vi "IT7800 Driver Test.vi"() -> ()   [LabVIEW 2025]
uses:
  <vilib>/Platform/TimedLoop/XDataNode/timing_clust.ctl
  <vilib>/Platform/TimedLoop/XDataNode/nitl_modes.ctl
  <vilib>/Platform/TimedLoop/XDataNode/wakeup.ctl
  TypeDefs/CMD - Control.ctl
  <vilib>/Platform/TimedLoop/XDataNode/XDataNode.xnode
  <vilib>/Platform/TimedLoop/XDataNode/XDNodeRunTimeDep.lvlib
  <instrlib>/IT7800/IT7800.lvlib
panel:
  in  "CLR Error":bool
  out "Error":string
  in  "Tabs":enum32{"Testing", "Commands"}(tab)
  out "ValRead":bool
  in  "ReadInfo":bool
  in  "Command":T1(ring)
  in  "Write":bool
  in  "Parameter":dbl=50.0
  out "Output ON":bool
  out "Phase Config":string="-"
  in  "Read":bool=TRUE
  out "PSU Values":T2
  out "IT7800 Info":T3
  out "PSU Values 3PH":T4
  in  "String":string="FETC:VOLT?;\\s:FETC:FREQ?;\\s:FETC:CURR?;\\s:FETC:CURR:CFAC?;\\s:FETC:LTLV?\\sBA\n\nFETC:POW:REAL?;\\sPOW:APP?;\\s:FETC:POW:REAC?;\\sPOW:PFAC?\n\nFETC:WHO:ACT:POS?;\\s:FETC:WHO:ACT:NEG?"
  in  "SendCMD":bool
  out "Response":string
  in  "Request":string="FETC:VOLT?; :FETC:FREQ?"
  out "Open string":string
  in  "Exit":bool
  out "COM":bool
  in  "Close COM":bool
  in  "Open COM":bool
  in  "PSU Address":refnum<visa-resource-name>="192.168.0.252"
  # "Note: Change pase configuration only when output OFF"
  # "Note: In 3phase system PSU values are averages from 3Phases"
  # "Other examples used in software..."
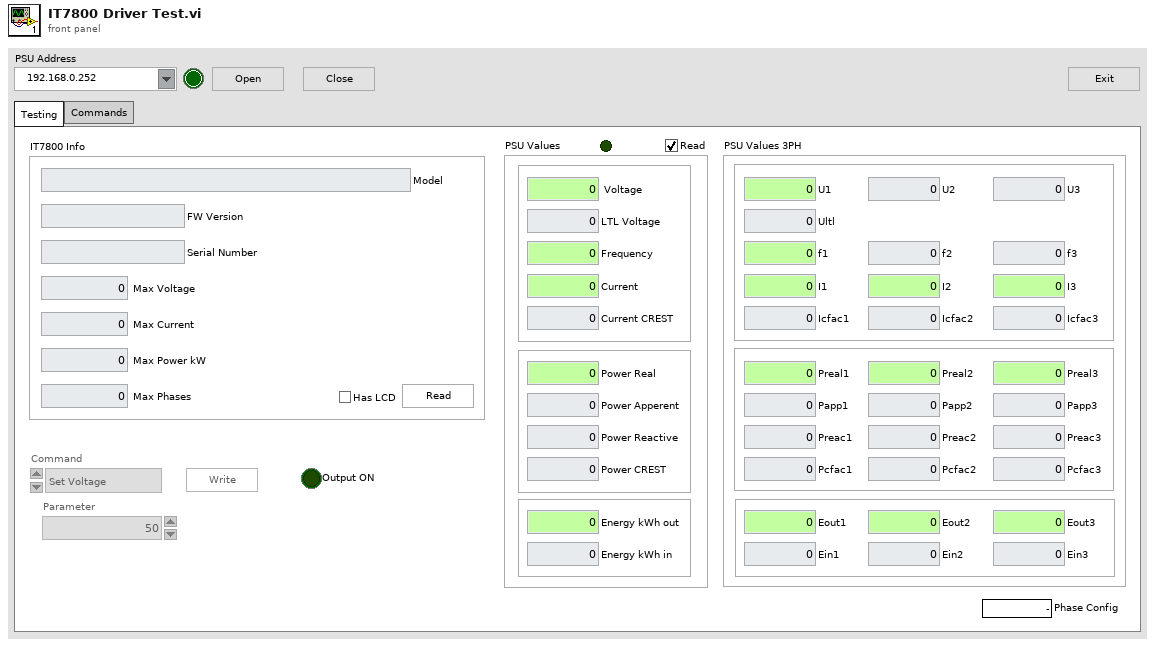
[diagram p1: front panel]
types:
  T1 = enum16{"Set Voltage", "Set Frequency", "Set to 1Phase", "Set to 3Phase", "Set to Split Phase", "Output ON", "Output OFF"}
  T2 = cluster{"Voltage":dbl, "LTL Voltage":dbl, "Current":dbl, "Current CREST":dbl, "Power Real":dbl, "Power Apperent":dbl, "Power Reactive":dbl, "Power CREST":dbl, "Energy kWh out":dbl, "Energy kWh in":dbl, "Frequency":dbl}
  T3 = cluster{"Model":string, "FW Version":string, "Serial Number":string, "Max Voltage":dbl, "Max Current":dbl, "Max Power kW":dbl, "Max Phases":u8, "Has LCD":bool}
  T4 = cluster{"U1":dbl, "U2":dbl, "U3":dbl, "Ultl":dbl, "f1":dbl, "f2":dbl, "f3":dbl, "I1":dbl, "I2":dbl, "I3":dbl, "Icfac1":dbl, "Icfac2":dbl, "Icfac3":dbl, "Preal1":dbl, "Preal2":dbl, "Preal3":dbl, "Papp1":dbl, "Papp2":dbl, "Papp3":dbl, "Preac1":dbl, "Preac2":dbl, "Preac3":dbl, "Pcfac1":dbl, "Pcfac2":dbl, "Pcfac3":dbl, "Eout1":dbl, "Eout2":dbl, "Eout3":dbl, "Ein1":dbl, "Ein2":dbl, "Ein3":dbl}
  T5 = enum32{"invalid app kind", "Development System", "Run Time System", "Student Edition", "Embedded LabVIEW", "Evaluation", "Custom"}
  T6 = enum8{"Enabled", "Disabled", "Disabled and Grayed Out"}
  T7 = typedef "XDNodeRunTimeDep.lvlib/timing_clust.ctl" = cluster{"Expected End [f-1]":u64, "Actual End [f-1]":u64, "Finished Late? [f-1]":bool, "Expected End [i-1]":u64, "Actual End [i-1]":u64, "Finished Late? [i-1]":bool, "Expected Start [i]":u64, "Actual Start [i]":u64, "Expected Start [f]":u64, "Actual Start [f]":u64, "Source Name":string, "Structure Name":string, "Period":i64, "Deadline":i64, "Offset":i64, "Start":i64, "Priority":i32, "Timeout":i32, "Mode":T8, "Wakeup Reason":T9, "Error":errorcluster, "Source Type":string, "Secondary Source Type":string, "Global End Time":u64, "Global Start Time":u64, "Frame Duration":u64, "Iteration Duration":u64, "Assigned CPU":i32, "I/O Scan Engine Mode":u32}
  T8 = typedef "XDNodeRunTimeDep.lvlib/nitl_modes.ctl" = enum32{"No Change", "Process missed periods, maintain original phase", "Discard missed periods, maintain original phase", "Process missed periods, ignore original phase", "Discard missed periods, ignore original phase"}
  T9 = typedef "XDNodeRunTimeDep.lvlib/wakeup.ctl" = enum32{"Normal", "Aborted", "Asynchronous wakeup", "Timing source error", "Timed loop error", "Timeout"}
  T10 = typedef "CMD - Control.ctl" = enum16{"Voltage", "Frquency", "Set Phases", "Output", "Measure Rate"}
  T11 = cluster{"Basic  quantities":bool, "Power":bool, "Energy":bool}
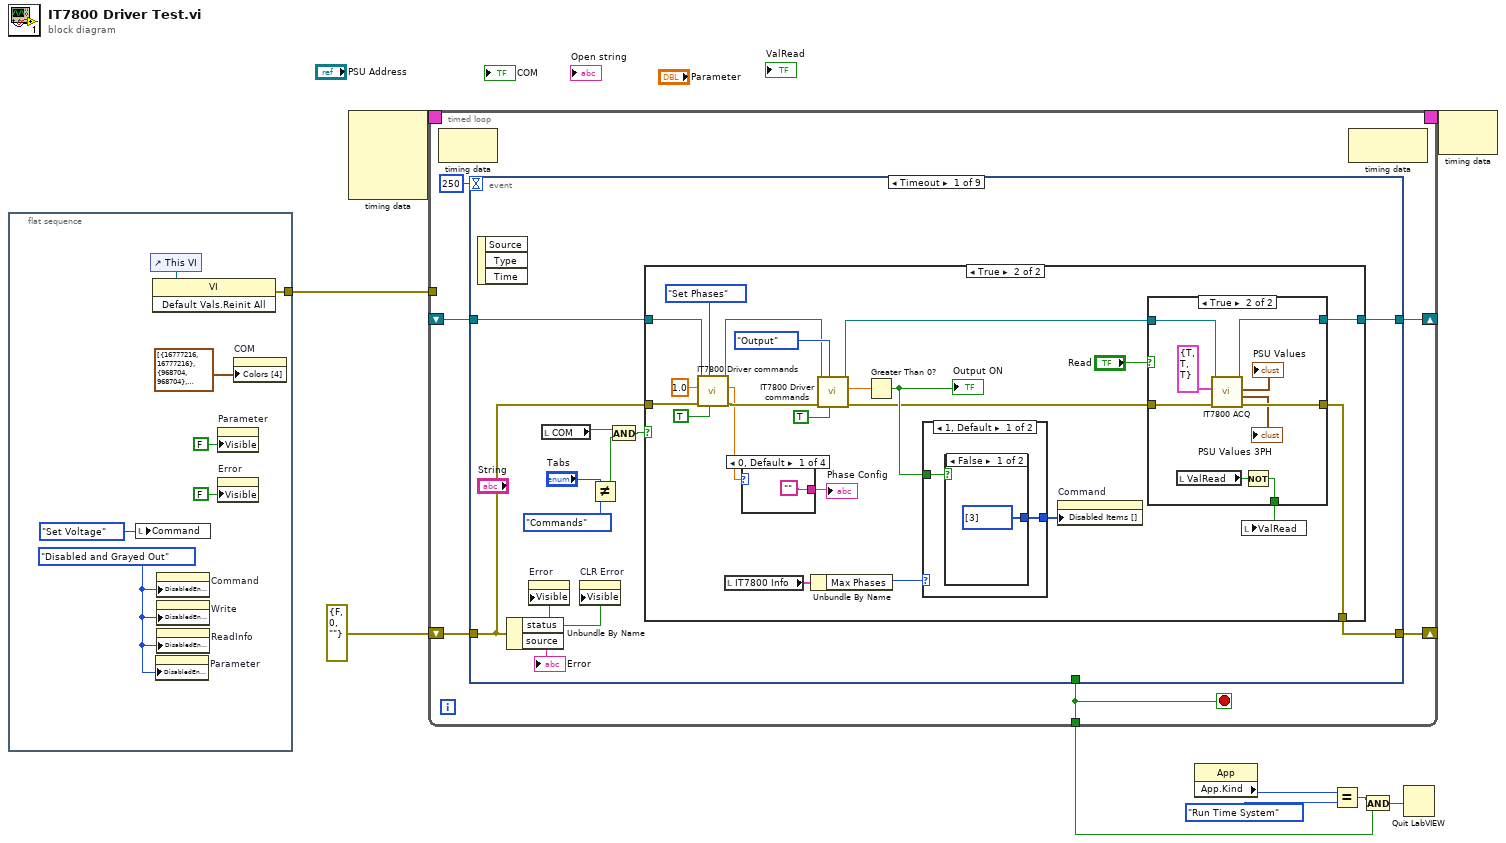
[diagram p0: block diagram]
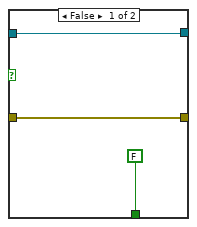
[diagram p3: hidden frame]
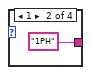
[diagram p4: hidden frame]
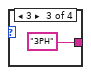
[diagram p5: hidden frame]
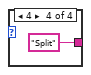
[diagram p6: hidden frame]
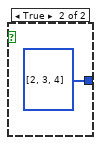
[diagram p7: hidden frame]
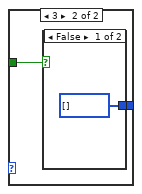
[diagram p8: hidden frame]
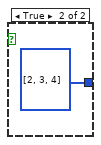
[diagram p9: hidden frame]
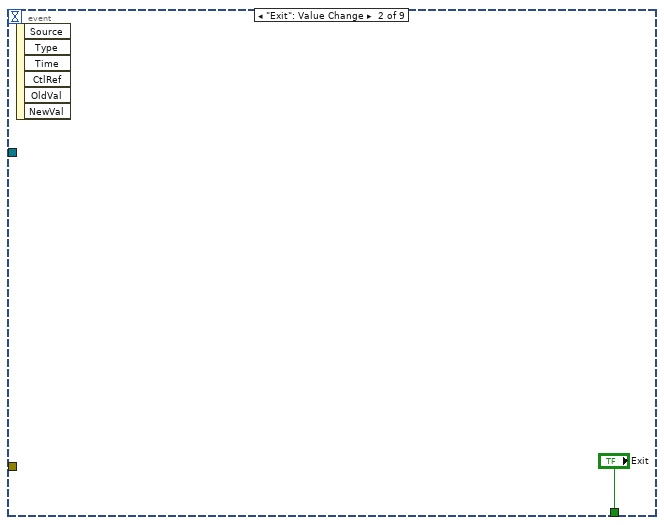
[diagram p10: hidden frame]
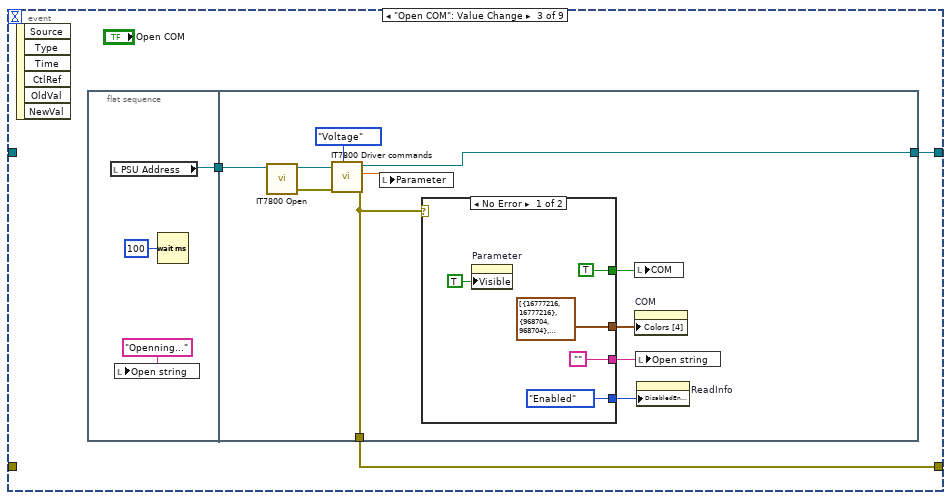
[diagram p11: hidden frame]
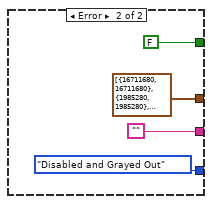
[diagram p12: hidden frame]
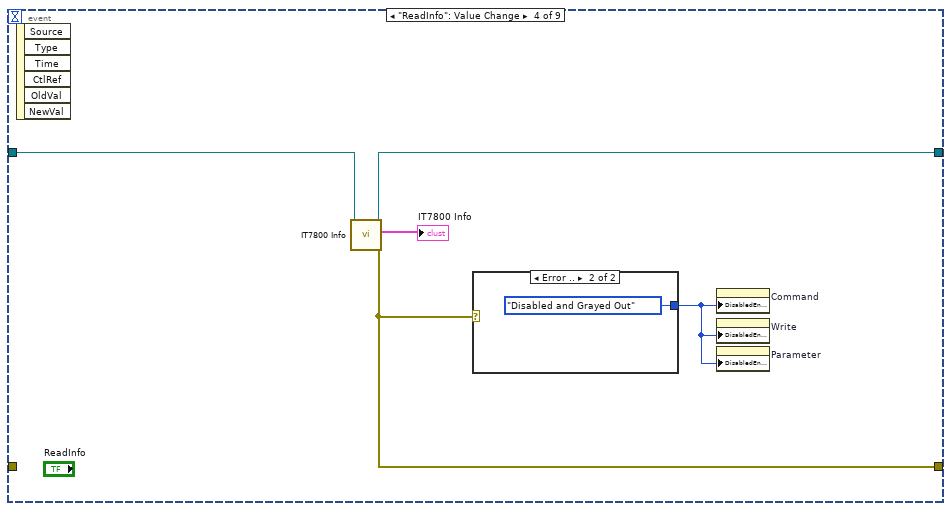
[diagram p13: hidden frame]
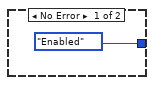
[diagram p14: hidden frame]
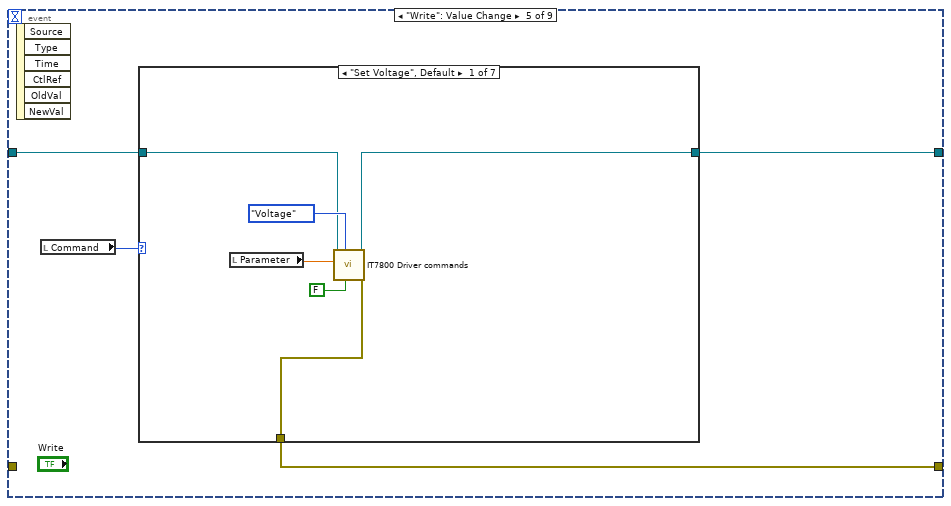
[diagram p15: hidden frame]
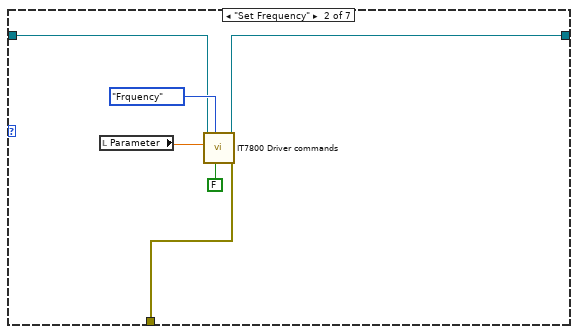
[diagram p16: hidden frame]
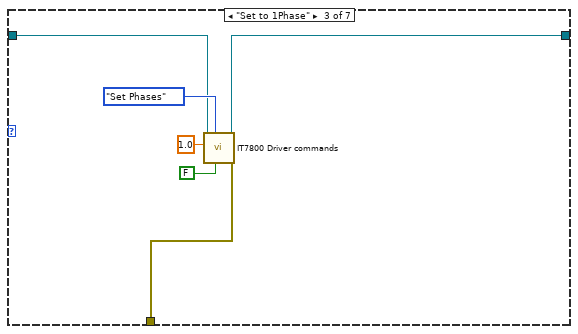
[diagram p17: hidden frame]
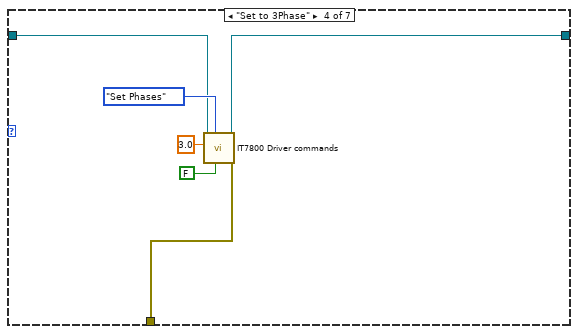
[diagram p18: hidden frame]
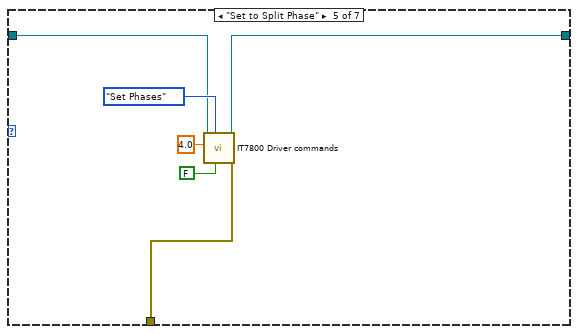
[diagram p19: hidden frame]
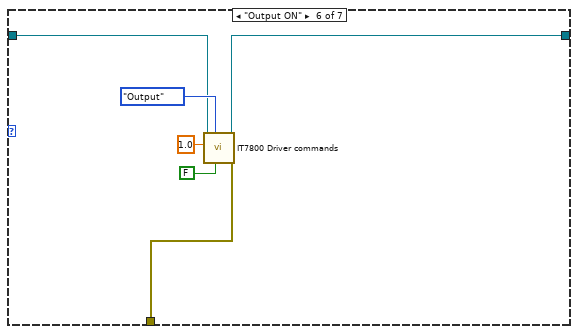
[diagram p20: hidden frame]
diagram:
  n1 = flat-sequence {
    tunnel: [w14] -> w2
    frame #0 {
      w10 = T6."Disabled and Grayed Out" ("Disabled")
      n2 = local write "Command"(T1."Set Voltage" ("Command")) -> ()
      n3 = control-ref of="This VI"() -> (w16:refnum<vi>)
      n4 = invoke class="VI" method="Default Vals.Reinit All"(reference=w16) -> (error out=w14:errorcluster)  [unwired: 2 in, 2 out]
      n5 = property on="Parameter" class="DigNum (strict)"("DisabledEnum"=w10) -> ()  [unwired: 2 in, 2 out]
      n6 = property on="Command" class="Enum (strict)"("DisabledEnum"=w10) -> ()  [unwired: 2 in, 2 out]
      n7 = property on="Write" class="Bool"("DisabledEnum"=w10) -> ()  [unwired: 2 in, 2 out]
      n8 = property on="ReadInfo" class="Bool"("DisabledEnum"=w10) -> ()  [unwired: 2 in, 2 out]
      n9 = property on="Parameter" class="DigNum (strict)"("Visible"=FALSE) -> ()  [unwired: 2 in, 2 out]
      n10 = property on="Error" class="Str"("Visible"=FALSE) -> ()  [unwired: 2 in, 2 out]
      n11 = property on="COM" class="Bool (strict)"("Colors [4]"=cluster{u32, u32}[] [{16777216, 16777216}, {968704, 968704}, {16777216, 16777216}, {484352, 484352}]) -> ()  [unwired: 2 in, 2 out]
    }
  }
  n12 = node-c288() -> (w9:T7)  [unwired: 4 in]
  n13 = timed-loop {
    timing: w9 -> [_]
    timing-out: [_] -> w8
    tunnel: [w22] -> w3
    tunnel: w2 -> [_]
    shift-right: [w17] -> _
    shift-left: _ -> [w21]
    shift-right: [w19] -> _
    shift-left: errorcluster {"status"=FALSE, "code"=0, "source"=""} ("error out") -> [w18]
    stop <- w22 stop-if-true
    n14 = node-c288() -> ()  [unwired: 1 in, 1 out]
    n15 = event shown="[0] Timeout" {
      selector: _ -> [_ _ _ _ _ _ _ _ _]
      dyn-events: _ -> [_ _ _ _ _ _ _ _ _]
      timeout: 250 -> [_ _ _ _ _ _ _ _ _]
      tunnel: [_ "Exit" _ _ _ _ _ _ _] -> w22
      tunnel: w21 -> [w33 _ _ w113 w118 w163 w193 w195 w204]
      tunnel: [w29 _ w83 w110 w116 w162 w184 w196 w202] -> w19
      tunnel: w18 -> [w30 _ _ _ _ _ w192 w197 _]
      tunnel: [w32 _ w84 w111 w117 w164 w183 w195 _] -> w17
      event Timeout {
        n16 = event-data() -> ()  [unwired: 1 in, 3 out]
        n17 = Unbundle By Name(w30) -> ("status"=w23:bool, "source"=→"Error":string)
        n18 = property on="Error" class="Str"("Visible"=w23) -> ()  [unwired: 2 in, 2 out]
        n19 = local read "COM"() -> (w26:bool)
        n20 = property on="CLR Error" class="Bool"("Visible"=w23) -> ()  [unwired: 2 in, 2 out]
        n21 = Not Equal?(x="Tabs", y=enum32{"Testing", "Commands"}."Commands" ("Tabs")) -> (x != y?=w25:bool)
        n22 = And(x=w26, y=w25) -> (x .and. y?=w24:bool)
        n23 = case shown="True" w24 {
          tunnel: w33 -> [w35 w43]
          tunnel: [w35 w50] -> w32
          tunnel: w30 -> [w34 w40]
          tunnel: [w34 w47] -> w29
          frame False {
          }
          frame True {
            n24 = call "IT7800 Driver commands.vi"("Read"=TRUE, "Command"=CMD_-_Control."Set Phases", "error in"=w40, "Data Write"=1.0, "VISA in"=w43) -> ("error out"=w41:errorcluster, "Data Read"=w39:dbl, "VISA out"=w42:refnum<visa-resource-name>)  [unwired: 3 in, 1 out]
            n25 = local read "IT7800 Info"() -> (w53:T3)
            n26 = case shown="0, Default" w39 {
              tunnel: ["" "1PH" ("Phases") "3PH" ("Phases") "Split" ("Phases")] -> w38
              frame 0, Default {
              }
              frame 1 {
              }
              frame 3 {
              }
              frame 4 {
              }
            }
            "Phase Config" <- w38
            n27 = Unbundle By Name(w53) -> ("Max Phases"=w52:u8)
            n28 = call "IT7800 Driver commands.vi"("Read"=TRUE, "Command"=CMD_-_Control."Output", "error in"=w41, "VISA in"=w42) -> ("error out"=w48:errorcluster, "Data Read"=w55:dbl, "VISA out"=w51:refnum<visa-resource-name>)  [unwired: 4 in, 1 out]
            n29 = Greater Than 0?(x=w55) -> (x > 0?=w49:bool)
            "Output ON" <- w49
            n30 = case shown="1, Default" w52 {
              tunnel: w49 -> [w75 w79]
              tunnel: [w74 w78] -> w54
              frame 1, Default {
                n31 = case shown="False" w75 {
                  tunnel: [i32[] [3] ("Disabled Items []") i32[] [2, 3, 4] ("Disabled Items []")] -> w74
                  frame False {
                  }
                  frame True {
                  }
                }
              }
              frame 3 {
                n32 = case shown="False" w79 {
                  tunnel: [i32[] [] ("Disabled Items []") i32[] [2, 3, 4] ("Disabled Items []")] -> w78
                  frame False {
                  }
                  frame True {
                  }
                }
              }
            }
            n33 = property on="Command" class="Enum (strict)"("Disabled Items []"=w54) -> ()  [unwired: 2 in, 2 out]
            n34 = case shown="True" "Read" {
              tunnel: w51 -> [w60 w69]
              tunnel: [w60 w68] -> w50
              tunnel: w48 -> [w59 w67]
              tunnel: [w59 w66] -> w47
              tunnel: [FALSE w62] -> w36
              frame False {
              }
              frame True {
                n35 = local read "ValRead"() -> (w63:bool)
                n36 = call "IT7800 ACQ.vi"("error in"=w67, "Read selection"=T11 {"Basic  quantities"=TRUE, "Power"=TRUE, "Energy"=TRUE}, "VISA in"=w69) -> ("error out"=w66:errorcluster, "PSU Values 3PH"=→"PSU Values 3PH":T4, "PSU Values"=→"PSU Values":T2, "VISA out"=w68:refnum<visa-resource-name>)  [unwired: 5 in]
                n37 = Not(x=w63) -> (.not. x?=w62:bool)
              }
            }
            n38 = local write "ValRead"(w36) -> ()
          }
        }
      }
      event "Exit": Value Change {
        n39 = event-data() -> ()  [unwired: 1 in, 6 out]
      }
      event "Open COM": Value Change {
        n40 = event-data() -> ()  [unwired: 1 in, 6 out]
        n41 = flat-sequence {
          tunnel: [w87] -> w85
          tunnel: w85 -> [w99]
          tunnel: [w92] -> w84
          tunnel: [w90] -> w83
          frame #0 {
            n42 = local read "PSU Address"() -> (w87:refnum<visa-resource-name>)
            n43 = local write "Open string"("Openning..." ("Opene string")) -> ()
            n44 = Wait (ms)(milliseconds to wait=u32 100) -> ()  [unwired: 1 out]
          }
          frame #1 {
            n45 = call "IT7800 Open.vi"("IP Address"=w99) -> ("error out"=w91:errorcluster, "VISA out"=w93:refnum<visa-resource-name>)  [unwired: 9 in]
            n46 = call "IT7800 Driver commands.vi"("Command"=CMD_-_Control."Voltage", "error in"=w91, "VISA in"=w93) -> ("error out"=w90:errorcluster, "Data Read"=w94:dbl, "VISA out"=w92:refnum<visa-resource-name>)  [unwired: 5 in, 1 out]
            n47 = local write "Parameter"(w94) -> ()
            n48 = case shown="No Error" w90 {
              tunnel: [cluster{u32, u32}[] [{16777216, 16777216}, {968704, 968704}, {16777216, 16777216}, {484352, 484352}] ("Colors [4]") cluster{u32, u32}[] [{16711680, 16711680}, {1985280, 1985280}, {16777216, 16777216}, {484352, 484352}] ("Colors [4]")] -> w98
              tunnel: [TRUE ("COM") FALSE ("COM")] -> w97
              tunnel: ["" ""] -> w96
              tunnel: [T6."Enabled" ("Disabled") T6."Disabled and Grayed Out" ("Disabled")] -> w89
              frame No Error {
                n49 = property on="Parameter" class="DigNum (strict)"("Visible"=TRUE) -> ()  [unwired: 2 in, 2 out]
              }
              frame Error {
              }
            }
            n50 = local write "COM"(w97) -> ()
            n51 = property on="COM" class="Bool (strict)"("Colors [4]"=w98) -> ()  [unwired: 2 in, 2 out]
            n52 = local write "Open string"(w96) -> ()
            n53 = property on="ReadInfo" class="Bool"("DisabledEnum"=w89) -> ()  [unwired: 2 in, 2 out]
          }
        }
      }
      event "ReadInfo": Value Change {
        n54 = event-data() -> ()  [unwired: 1 in, 6 out]
        n55 = call "IT7800 Info.vi"("VISA in"=w113) -> ("error out"=w110:errorcluster, "IT7800 Info"=→"IT7800 Info":T3, "VISA out"=w111:refnum<visa-resource-name>)  [unwired: 8 in]
        n56 = case shown="Error .." w110 {
          tunnel: [T6."Enabled" ("Disabled") T6."Disabled and Grayed Out" ("Disabled")] -> w109
          frame No Error {
          }
          frame Error {
          }
        }
        n57 = property on="Command" class="Enum (strict)"("DisabledEnum"=w109) -> ()  [unwired: 2 in, 2 out]
        n58 = property on="Write" class="Bool"("DisabledEnum"=w109) -> ()  [unwired: 2 in, 2 out]
        n59 = property on="Parameter" class="DigNum (strict)"("DisabledEnum"=w109) -> ()  [unwired: 2 in, 2 out]
      }
      event "Write": Value Change {
        n60 = event-data() -> ()  [unwired: 1 in, 6 out]
        n61 = local read "Command"() -> (w119:T1)
        n62 = case shown="\"Set Voltage\", Default" w119 {
          tunnel: w118 -> [w124 w130 w136 w142 w148 w154 w160]
          tunnel: [w123 w129 w135 w141 w147 w153 w156] -> w117
          tunnel: [w120 w126 w132 w138 w144 w150 w157] -> w116
          frame "Set Voltage", Default {
            n63 = local read "Parameter"() -> (w122:dbl)
            n64 = call "IT7800 Driver commands.vi"("Read"=FALSE, "Command"=CMD_-_Control."Voltage", "Data Write"=w122, "VISA in"=w124) -> ("error out"=w120:errorcluster, "VISA out"=w123:refnum<visa-resource-name>)  [unwired: 4 in, 2 out]
          }
          frame "Set Frequency" {
            n65 = local read "Parameter"() -> (w128:dbl)
            n66 = call "IT7800 Driver commands.vi"("Read"=FALSE, "Command"=CMD_-_Control."Frquency", "Data Write"=w128, "VISA in"=w130) -> ("error out"=w126:errorcluster, "VISA out"=w129:refnum<visa-resource-name>)  [unwired: 4 in, 2 out]
          }
          frame "Set to 1Phase" {
            n67 = call "IT7800 Driver commands.vi"("Read"=FALSE, "Command"=CMD_-_Control."Set Phases", "Data Write"=1.0, "VISA in"=w136) -> ("error out"=w132:errorcluster, "VISA out"=w135:refnum<visa-resource-name>)  [unwired: 4 in, 2 out]
          }
          frame "Set to 3Phase" {
            n68 = call "IT7800 Driver commands.vi"("Read"=FALSE, "Command"=CMD_-_Control."Set Phases", "Data Write"=3.0, "VISA in"=w142) -> ("error out"=w138:errorcluster, "VISA out"=w141:refnum<visa-resource-name>)  [unwired: 4 in, 2 out]
          }
          frame "Set to Split Phase" {
            n69 = call "IT7800 Driver commands.vi"("Read"=FALSE, "Command"=CMD_-_Control."Set Phases", "Data Write"=4.0, "VISA in"=w148) -> ("error out"=w144:errorcluster, "VISA out"=w147:refnum<visa-resource-name>)  [unwired: 4 in, 2 out]
          }
          frame "Output ON" {
            n70 = call "IT7800 Driver commands.vi"("Read"=FALSE, "Command"=CMD_-_Control."Output", "Data Write"=1.0, "VISA in"=w154) -> ("error out"=w150:errorcluster, "VISA out"=w153:refnum<visa-resource-name>)  [unwired: 4 in, 2 out]
          }
          frame "Output OFF" {
            n71 = call "IT7800 Driver commands.vi"("Read"=FALSE, "Command"=CMD_-_Control."Output", "Data Write"=0.0, "VISA in"=w160) -> ("error out"=w157:errorcluster, "VISA out"=w156:refnum<visa-resource-name>)  [unwired: 4 in, 2 out]
          }
        }
      }
      event "Command": Value Change {
        n72 = event-data() -> ()  [unwired: 1 in, 6 out]
        n73 = case shown="\"Set Voltage\"" "Command" {
          tunnel: [TRUE ("Visible") TRUE ("Visible") FALSE ("Visible")] -> w165
          tunnel: w163 -> [w171 w175 w180]
          tunnel: [w170 w174 w180] -> w164
          tunnel: [w167 w173 errorcluster {"status"=FALSE, "code"=0, "source"=""} ("error out")] -> w162
          frame "Set Voltage" {
            n74 = call "IT7800 Driver commands.vi"("Command"=CMD_-_Control."Voltage", "VISA in"=w171) -> ("error out"=w167:errorcluster, "Data Read"=w168:dbl, "VISA out"=w170:refnum<visa-resource-name>)  [unwired: 6 in, 1 out]
            n75 = local write "Parameter"(w168) -> ()
          }
          frame "Set Frequency" {
            n76 = call "IT7800 Driver commands.vi"("Command"=CMD_-_Control."Frquency", "VISA in"=w175) -> ("error out"=w173:errorcluster, "Data Read"=w176:dbl, "VISA out"=w174:refnum<visa-resource-name>)  [unwired: 6 in, 1 out]
            n77 = local write "Parameter"(w176) -> ()
          }
          frame "Set to 1Phase", Default {
          }
        }
        n78 = property on="Parameter" class="DigNum (strict)"("Visible"=w165) -> ()  [unwired: 2 in, 2 out]
      }
      event "SendCMD": Value Change {
        n79 = event-data() -> ()  [unwired: 1 in, 6 out]
        n80 = Concatenate Strings("Request", "\n") -> (w189:string)
        n81 = VISA Write(VISA resource name=w193, write buffer=w189, error in (no error)=w192) -> (VISA resource name out=w188:refnum<visa-resource-name>, error out=w187:errorcluster)  [unwired: 1 out]
        n82 = VISA Read(VISA resource name=w188, byte count=u32 1024, error in (no error)=w187) -> (VISA resource name out=w182:refnum<visa-resource-name>, read buffer=→"Response":string, error out=w185:errorcluster)  [unwired: 1 out]
        n83 = call <instrlib>:"Error Query.vi"("error in"=w185, "VISA resource name"=w182) -> ("error out"=w184:errorcluster, "VISA resource name out"=w183:refnum<visa-resource-name>)  [unwired: 6 in, 2 out]
      }
      event "CLR Error": Value Change {
        n84 = event-data() -> ()  [unwired: 1 in, 6 out]
        n85 = case shown="True" "CLR Error" {
          tunnel: w197 -> [w199 _]
          tunnel: [w199 errorcluster {"status"=FALSE, "code"=0, "source"=""} ("error out")] -> w196
          frame False {
          }
          frame True {
          }
        }
      }
      event "Close COM": Value Change {
        n86 = event-data() -> ()  [unwired: 1 in, 6 out]
        n87 = local read "COM"() -> (w203:bool)
        n88 = case shown="False" w203 {
          tunnel: w204 -> [_ w208]
          tunnel: [errorcluster {"status"=FALSE, "code"=0, "source"=""} ("error out") w207] -> w202
          frame False {
          }
          frame True {
            n89 = local write "COM"(FALSE ("COM")) -> ()
            n90 = call "IT7800 Close.vi"("VISA in"=w208) -> ("error out"=w207:errorcluster)  [unwired: 9 in, 1 out]
          }
        }
        n91 = local write "ValRead"(FALSE ("ValRead")) -> ()
        n92 = property on="COM" class="Bool (strict)"("Colors [4]"=cluster{u32, u32}[] [{16777216, 16777216}, {968704, 968704}, {16777216, 16777216}, {484352, 484352}]) -> ()  [unwired: 2 in, 2 out]
      }
    }
    n93 = node-c288() -> ()  [unwired: 1 in, 1 out]
  }
  n94 = property class="App"() -> ("App.Kind"=w5:T5)  [unwired: 2 in, 2 out]
  n95 = Equal?(x=w5, y=T5."Run Time System" ("Application:Kind")) -> (x = y?=w7:bool)
  n96 = And(x=w7, y=w3) -> (x .and. y?=w4:bool)
  n97 = Quit LabVIEW(quit? (T)=w4) -> ()
  n98 = node-c288(w8) -> ()  [unwired: 1 out]
